vi "Disable Ports already taken.vi"(8 "error in (no error)":errorcluster, 9 "Values":u16[](array[numeric]), 10 "COM Port numbers taken":i32[](array[numeric]), 11 "Ctrl References":refnum<vi>[](array[refnum])) -> (0 "error out":errorcluster)   [LabVIEW 2011]
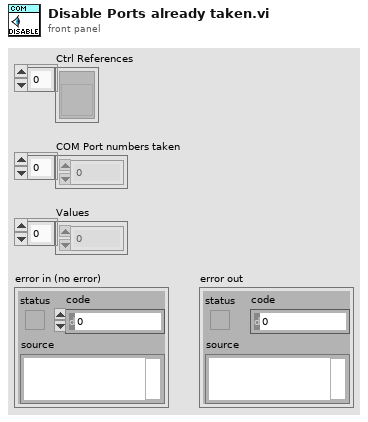
[diagram p1: front panel]
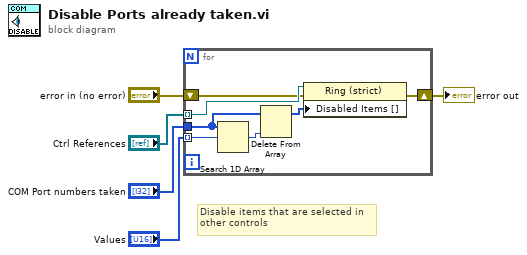
[diagram p0: block diagram]
diagram:
  # "Disable items that are selected in \nother controls"
  n1 = for {
    tunnel: "Ctrl References" -> [w12] mode=indexing
    shift-right: [w11] -> w5
    shift-left: "error in (no error)" -> [w10]
    tunnel: "COM Port numbers taken" -> [w8]
    tunnel: "Values" -> [w9] mode=indexing
    n2 = Search 1D Array(1D array=w8, element=w9) -> (index of element=w7:i32)  [unwired: 1 in]
    n3 = Delete From Array(array=w8, index=w7) -> (array with subset deleted=w6:i32[])  [unwired: 1 in, 1 out]
    n4 = property class="Ring (strict)"(reference=w12, error in=w10, "Disabled Items []"=w6) -> (error out=w11:errorcluster)  [unwired: 1 out]
  }
  "error out" <- w5
